vi "Remove Empty Rows.vi"(11 "Array in":string[][](array[string])) -> (3 "Array out":string[][](array[string]))   [LabVIEW 2015]
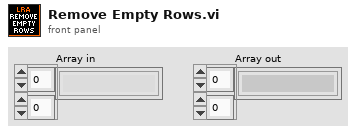
[diagram p1: front panel]
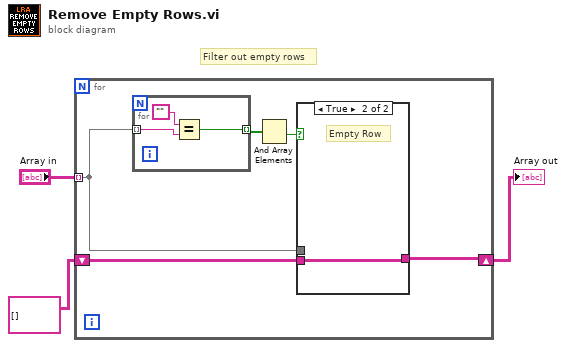
[diagram p0: block diagram]
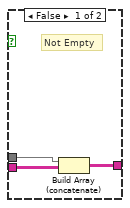
[diagram p2: hidden frame]
diagram:
  # "Filter out empty rows"
  n1 = for {
    tunnel: "Array in" -> [w4] mode=indexing
    shift-right: [w5] -> w3
    shift-left: string[][] [] -> [w6]
    n2 = for {
      tunnel: w4 -> [w15] mode=indexing
      tunnel: [w13] -> w8 mode=indexing
      n3 = Equal?(x="", y=w15) -> (x = y?=w13:bool)
    }
    n4 = And Array Elements(Boolean array=w8) -> (logical AND=w7:bool)
    n5 = case shown="True" w7 {
      tunnel: w6 -> [w11 w12]
      tunnel: [w10 w12] -> w5
      tunnel: w4 -> [w9 _]
      frame False {
        # "Not Empty"
        n6 = Build Array (concatenate)(w9, w11) -> (w10:string[][])
      }
      frame True {
        # "Empty Row"
      }
    }
  }
  "Array out" <- w3
